vi "LINE_v1.vi"() -> ()   [LabVIEW 2010]
uses:
  <vilib>/express/express arith-compare/Formula/XNode/ExpressFormulaBlockNode.xnode
panel:
  in  "x-dist":u32
  in  "Motor GPIB":u8=6
  in  "speed":u16
  in  "y-dist":u32
  in  "Current (mA)":dbl
  in  "Laser GPIB":u8=10 max=100
  out "Dummy":string
  # "LINE<space>[Displacement]<space>[Speed]<space>[Current]"
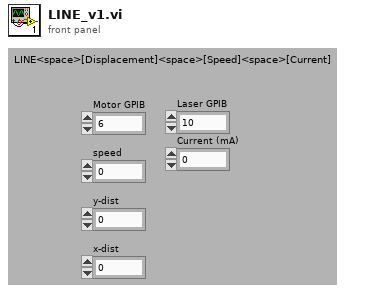
[diagram p1: front panel]
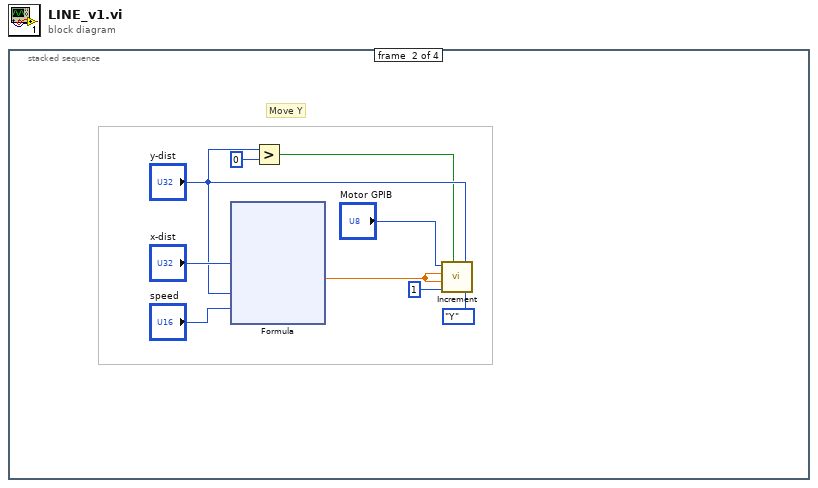
[diagram p0: block diagram]
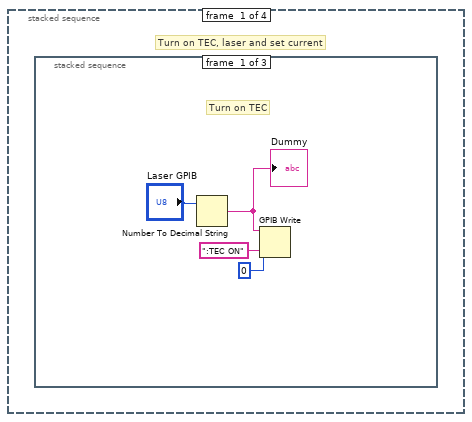
[diagram p2: hidden frame]
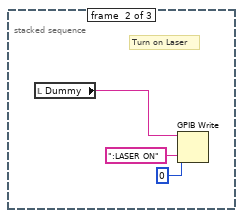
[diagram p3: hidden frame]
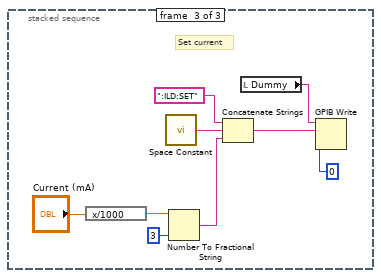
[diagram p4: hidden frame]
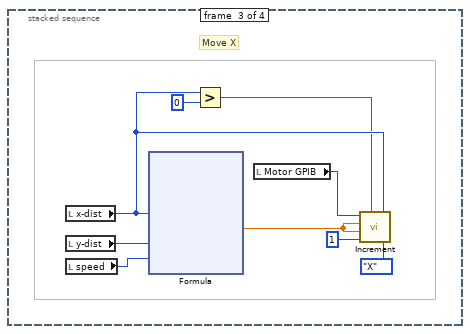
[diagram p5: hidden frame]
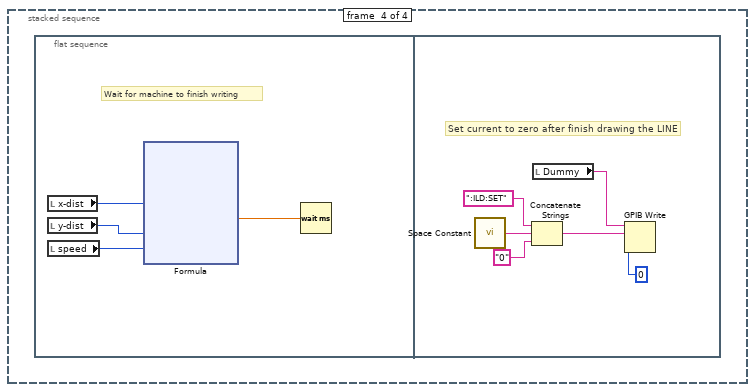
[diagram p6: hidden frame]
diagram:
  n1 = stacked-sequence {
    frame #0 {
      # "Turn on TEC, laser and set current"
      n2 = stacked-sequence {
        frame #0 {
          # "Turn on TEC"
          n3 = Number To Decimal String(number="Laser GPIB") -> (decimal integer string=w1:string)  [unwired: 1 in]
          "Dummy" <- w1
          n4 = GPIB Write(0:w1, 1:":TEC ON" ("data"), 2:i16 0 ("mode (0)")) -> ()  [unwired: 2 in, 2 out]
        }
        frame #1 {
          # "Turn on Laser"
          n5 = local read "Dummy"() -> (w5:string)
          n6 = GPIB Write(0:w5, 1:":LASER ON" ("data"), 2:i16 0 ("mode (0)")) -> ()  [unwired: 2 in, 2 out]
        }
        frame #2 {
          # "Set current"
          n7 = expression code="x/1000"("Current (mA)") -> (w12:dbl)
          n8 = call <vilib>:"Space Constant.vi"() -> ("String"=w14:string)
          n9 = Number To Fractional String(number=w12, precision (6)=i16 3) -> (F-format string=w9:string)  [unwired: 2 in]
          n10 = Concatenate Strings(":ILD:SET", w14, w9) -> (w13:string)
          n11 = local read "Dummy"() -> (w8:string)
          n12 = GPIB Write(0:w8, 1:w13, 2:i16 0 ("mode (0)")) -> ()  [unwired: 2 in, 2 out]
        }
      }
    }
    frame #1 {
      # "Move Y"
      n13 = xnode "Formula"("X1"="x-dist", "X2"="y-dist", "X3"="speed") -> ("Result"=w20:dbl)  [unwired: 1 in, 1 out]
      n14 = Greater?(x="y-dist", y=u32 0) -> (0:w17:bool)
      n15 = call "Increment.vi"("GPIB_Addr"="Motor GPIB", "F Speed"=w20, "L Speed"=w20, "Rate"=u16 1, "CCW 3"=w17, "Distance"="y-dist", "Axis"=enum16{"X", "Y", "Z", "U", "V", "W"}."Y") -> ()
    }
    frame #2 {
      # "Move X"
      n16 = local read "x-dist"() -> (w40:u32)
      n17 = local read "y-dist"() -> (w43:u32)
      n18 = local read "speed"() -> (w42:u16)
      n19 = xnode "Formula"("X1"=w40, "X2"=w43, "X3"=w42) -> ("Result"=w44:dbl)  [unwired: 1 in, 1 out]
      n20 = Greater?(x=w40, y=u32 0) -> (0:w38:bool)
      n21 = local read "Motor GPIB"() -> (w41:u8)
      n22 = call "Increment.vi"("GPIB_Addr"=w41, "F Speed"=w44, "L Speed"=w44, "Rate"=u16 1, "CCW 3"=w38, "Distance"=w40, "Axis"=enum16{"X", "Y", "Z", "U", "V", "W"}."X") -> ()
    }
    frame #3 {
      n23 = flat-sequence {
        frame #0 {
          # "Wait for machine to finish writing"
          n24 = local read "x-dist"() -> (w62:u32)
          n25 = local read "y-dist"() -> (w61:u32)
          n26 = local read "speed"() -> (w60:u16)
          n27 = xnode "Formula"("X1"=w62, "X2"=w61, "X3"=w60) -> ("Result"=w59:dbl)  [unwired: 1 in, 1 out]
          n28 = Wait (ms)(milliseconds to wait=w59) -> ()  [unwired: 1 out]
        }
        frame #1 {
          # "Set current to zero after finish drawing the LINE"
          n29 = call <vilib>:"Space Constant.vi"() -> ("String"=w78:string)
          n30 = Concatenate Strings(":ILD:SET", w78, "0" ("string")) -> (w77:string)
          n31 = local read "Dummy"() -> (w75:string)
          n32 = GPIB Write(0:w75, 1:w77, 2:i16 0 ("mode (0)")) -> ()  [unwired: 2 in, 2 out]
        }
      }
    }
  }
